vi "Construct.vi"(8 "Error in (no error)":errorcluster, 10 "Buffer":T1=50) -> (0 "Error out":errorcluster, 3 "LogWriterMock out":refnum<class "LogWriterMock.lvclass">)   [LabVIEW 2011, in "LogWriterMock.lvclass"]
uses:
  LogWriterMock.lvclass
  Log/Buffer.ctl
  LogWriterMock.lvclass/LogWriterMock.ctl
  Log/Log.lvclass
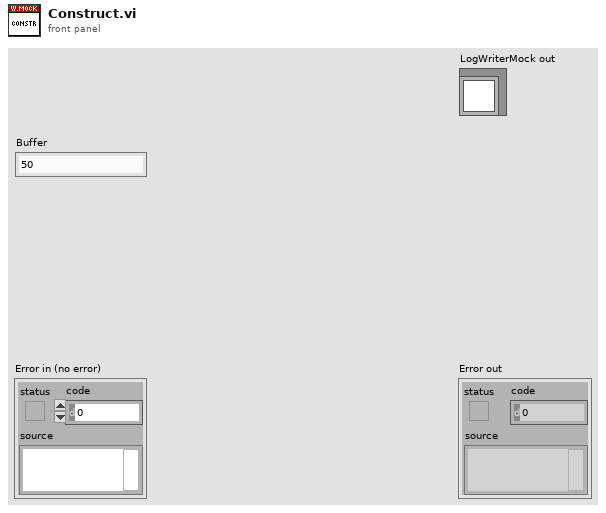
[diagram p1: front panel]
types:
  T1 = typedef "Log.lvclass/Buffer.ctl" = u32
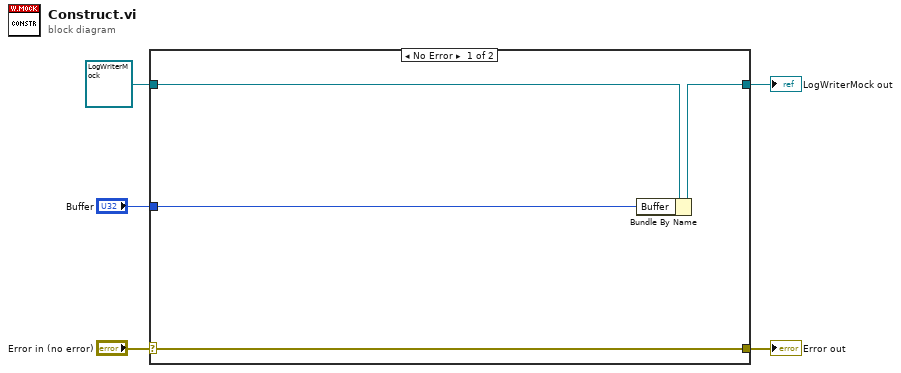
[diagram p0: block diagram]
diagram:
  n1 = case shown="No Error" "Error in (no error)" {
    selector: "Error in (no error)" -> [w9 w11]
    tunnel: [w9 w11] -> w4
    tunnel: [w6 w10] -> w3
    tunnel: refnum<class "LogWriterMock.lvclass"> refnum ("LogWriterMock in") -> [w7 w10]
    tunnel: "Buffer" -> [w8 _]
    frame No Error {
      n2 = Bundle By Name(cluster=w7, "Buffer"=w8) -> (w6:refnum<class "LogWriterMock.lvclass">)
    }
    frame Error {
    }
  }
  "Error out" <- w4
  "LogWriterMock out" <- w3
